vi "excel write zf.vi"() -> ()   [LabVIEW 2021]
uses:
  <vilib>/Utility/file.llb/Write Delimited Spreadsheet (string).vi
panel:
  in  "Array":cluster{"Value 1":dbl, "Message":string}[](array[cluster])
  # "Data write to Excel from LabView"
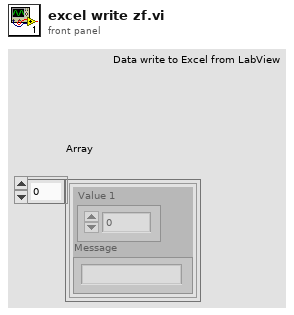
[diagram p1: front panel]
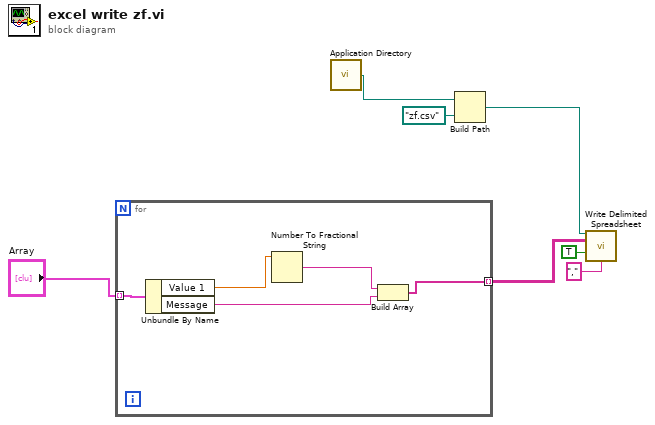
[diagram p0: block diagram]
diagram:
  n1 = for {
    tunnel: "Array" -> [w12] mode=indexing
    tunnel: [w10] -> w2 mode=indexing
    n2 = Unbundle By Name(w12) -> ("Value 1"=w9:dbl, "Message"=w11:string)
    n3 = Number To Fractional String(number=w9) -> (F-format string=w8:string)  [unwired: 3 in]
    n4 = Build Array(w8, w11) -> (w10:string[])
  }
  n5 = call <vilib>:"Application Directory.vi"() -> ("Application Directory"=w5:path)
  n6 = Build Path(base path=w5, name or relative path=path "zf.csv") -> (appended path=w4:path)
  n7 = call-poly <vilib>:"Write Delimited Spreadsheet.vi"("file path (dialog if empty)"=w4, "2D data"=w2, "append to file? (new file:F)"=TRUE, "delimiter (\\t)"="," ("delimiter (\\t)")) -> ()  [unwired: 10 in, 2 out]
